vi "Set Oil Pump RPM.vi"(0 "Session Handle in":T1, 5 "RPM":dbl format="%#_13g", 11 "error in (no error)":errorcluster) -> (4 "Session Handle out":T1, 6 "Failure Reason":string, 8 "Success?":bool, 15 "error out":errorcluster)   [LabVIEW 2015, in "Oil.lvclass"]
uses:
  Oil.lvclass
  Typedefs/Session Handle.ctl
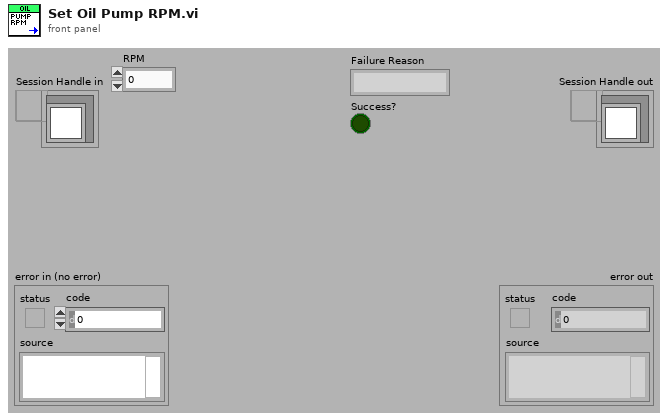
[diagram p1: front panel]
types:
  T1 = typedef "Oil.lvclass/Session Handle.ctl" = refnum<data-value>
  T2 = typedef "XNET Frame CAN.ctl" = cluster{"timestamp":timestamp, "payload":u8[], "identifier":u32, "type":T3, "extended?":bool, "echo?":bool}
  T3 = typedef "XNET Frame Type CAN.ctl" = u8
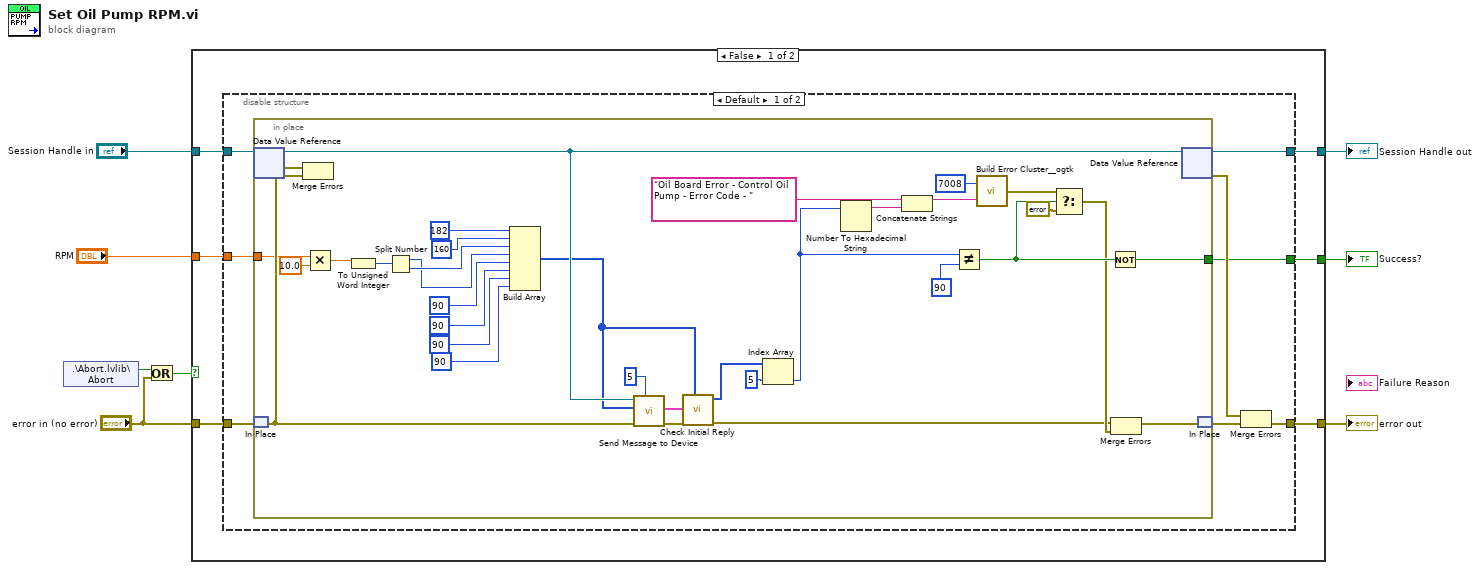
[diagram p0: block diagram]
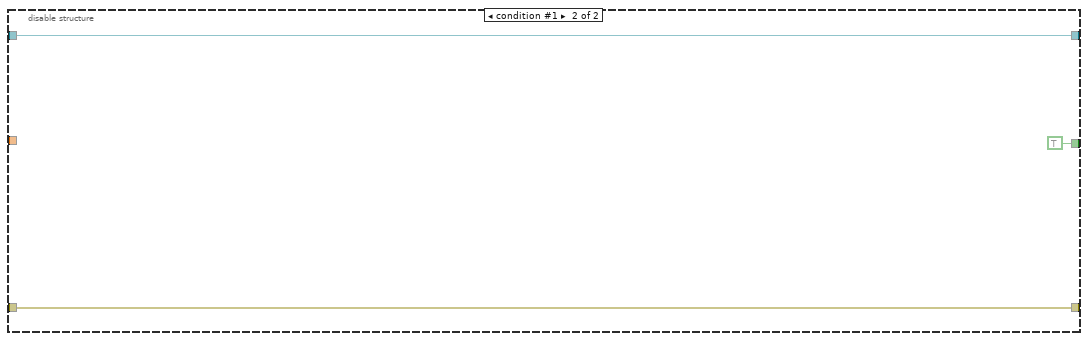
[diagram p2: hidden frame]
diagram:
  n1 = shared-variable ".\\Abort.lvlib\\Abort"() -> (w5:bool)  [unwired: 1 in, 1 out]
  n2 = Or(x=w5, y="error in (no error)") -> (x .or. y?=w4:bool)
  n3 = case shown="False" w4 {
    tunnel: "Session Handle in" -> [w14 w61]
    tunnel: [w13 w61] -> w7
    tunnel: [w12 w60] -> w6
    tunnel: "error in (no error)" -> [w11 w60]
    tunnel: [w10 _] -> w2
    tunnel: "RPM" -> [w9 _]
    frame False {
      n4 = disable-structure shown="Default" {
        disable-tunnel: w14 -> [w22 w59]
        disable-tunnel: [w21 w59] -> w13
        disable-tunnel: [w18 w57] -> w12
        disable-tunnel: w11 -> [w17 w57]
        disable-tunnel: [w16 TRUE] -> w10
        disable-tunnel: w9 -> [w15 _]
        frame condition #0 (active) {
          n5 = in-place {
            in-place-border: [w39] -> w16
            in-place-border: w15 -> [w28]
            n6 = in-place-dvr #1(w22) -> (w52:refnum<class "Oil.lvclass">, w56:errorcluster)
            n7 = in-place-match #2(w17) -> (w53:errorcluster)
            n8 = Merge Errors(w53, w56) -> ()  [unwired: 1 out]
            n9 = Multiply(x=w28, y=10.0) -> (x*y=w26:dbl)
            n10 = To Unsigned Word Integer(number=w26) -> (unsigned 16bit integer=w25:u16)
            n11 = Split Number(x=w25) -> (hi(x)=w23:u8, lo(x)=w24:u8)
            n12 = Build Array(u8 182 ("new element/subarray"), u8 160 ("new element/subarray"), w24, w23, u8 90 ("new element/subarray"), u8 90 ("new element/subarray"), u8 90 ("new element/subarray"), u8 90 ("new element/subarray")) -> (w50:u8[])
            n13 = call "Send Message to Device.vi"("Number of Retries"=5, "error in (no error)"=w53, "payload"=w50, "CAN Comm In"=w52) -> ("error out"=w36:errorcluster, "Reply"=w54:T2[])  [unwired: 5 in, 1 out]
            n14 = call "Check Initial Reply.vi"("Write Message"=w50, "error in (no error)"=w36, "Reply"=w54) -> ("error out"=w35:errorcluster, "Data Packet 2"=w51:u8[])  [unwired: 5 in, 2 out]
            n15 = Index Array(array=w51, index=5) -> (element=w40:u8)
            n16 = Number To Hexadecimal String(2:w40) -> (0:w42:string)  [unwired: 1 in]
            n17 = Concatenate Strings("Oil Board Error - Control Oil Pump - Error Code - " ("string"), w42) -> (w47:string)
            n18 = Not Equal?(x=w40, y=u8 90 ("new element/subarray")) -> (x != y?=w43:bool)
            n19 = call <userlib>:"Build Error Cluster__ogtk.vi"("String to Prepend to source (\"\")"=w47, "code"=7008) -> ("error out"=w45:errorcluster)
            n20 = Select(t=w45, s=w43, f=errorcluster {"status"=FALSE, "code"=0, "source"=""}) -> (s? t:f=w38:errorcluster)
            n21 = Not(x=w43) -> (.not. x?=w39:bool)
            n22 = Merge Errors(w35, w38) -> (w37:errorcluster)
            n23 = in-place-dvr #1(w52) -> (w21:T1, w19:errorcluster)
            n24 = in-place-match #2(w37) -> (w20:errorcluster)
          }
          n25 = Merge Errors(w19, w20) -> (w18:errorcluster)
        }
        frame condition #1 {
        }
      }
    }
    frame True {
    }
  }
  "Session Handle out" <- w7
  "error out" <- w6
  "Success?" <- w2
